vi "Create.vi"(8 "error in (no error)":errorcluster) -> (0 "error out":errorcluster, 3 "TestCase out":refnum<class "TestCase.lvclass">)   [LabVIEW 2011, in "DoNotWaitOnTestComplete.lvclass"]
uses:
  DoNotWaitOnTestComplete.lvclass
  Classes/TestCase/TestCase.lvclass
panel:
  # "Copyright © 2007 James Kring, Inc. All rights reserved.\n\nAuthor: Jim Kring [jim.kring@jameskring.com]\n\nThis library is provided \"AS IS\" ,WITHOUT WARRANTIES OR \nCONDITIONS OF ANY KIND, either express or implied.\n\nJames Kring, Inc. -- http://www.jameskring.com"
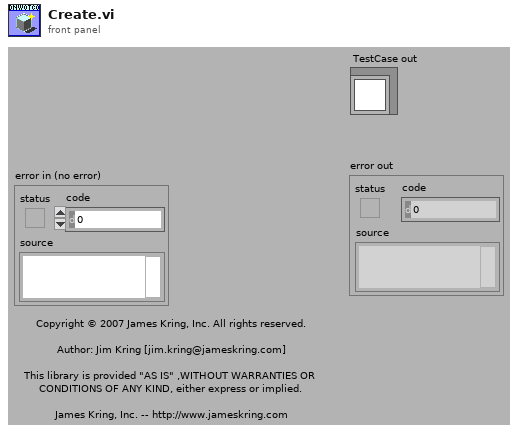
[diagram p1: front panel]
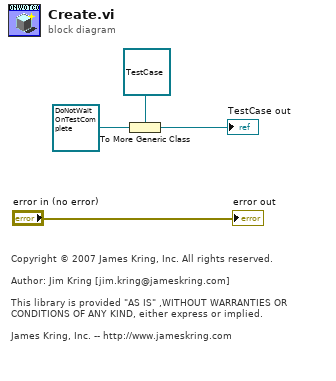
[diagram p0: block diagram]
diagram:
  # "Copyright © 2007 James Kring, Inc. All rights reserved.\n\nAuthor: Jim Kring [jim.kring@jameskring.com]\n\nThis library is provided \"AS IS\" ,WITHOUT WARRANTIES OR \nCONDITIONS OF ANY KIND, either express or implied.\n\nJames Kring, Inc. -- http://www.jameskring.com"
  n1 = To More Generic Class(target class=refnum<class "TestCase.lvclass"> refnum ("TestCase.lvclass"), reference=refnum<class "DoNotWaitOnTestComplete.lvclass"> refnum ("MyFirstTest.lvclass")) -> (generic class reference=→"TestCase out":refnum<class "TestCase.lvclass">)
  "error out" <- "error in (no error)"
